vi "Run Step.vi"(8 "error in (no error)":errorcluster, 9 "result allocation":T1, 10 "parameters":T1, 11 "Step in":refnum<class "Step.lvclass">) -> (0 "error out":errorcluster, 1 "results":T1, 2 "parameter allocation":T1, 3 "Step out":refnum<class "Step.lvclass">)   [LabVIEW 2015, in "Step.lvclass"]
uses:
  Step.lvclass
  <vilib>/NI/Tag Bus/table/data table.ctl
  StepState.ctl
  Step State Enum.ctl
  Step Flow Control.ctl
  Step.lvclass/Step.ctl
  <vilib>/NI/Tag Bus/table/data table.lvlib
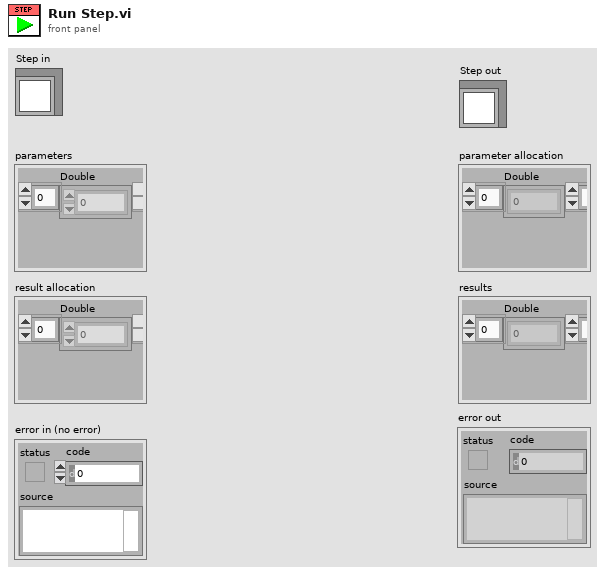
[diagram p1: front panel]
types:
  T1 = typedef "tag bus.lvlib/data table.lvlib/data table.ctl" = cluster{"Double":dbl[], "Single":sgl[], "I64":i64[], "I32":i32[], "I16":i16[], "I8":i8[], "U64":u64[], "U32":u32[], "U16":u16[], "U8":u8[], "Boolean":bool[], "String":string[], "Array of Double":cluster{"DBL Array":dbl[]}[], "Array of Single":cluster{"SGL Array":sgl[]}[], "Array of I64":cluster{"I64 Array":i64[]}[], "Array of I32":cluster{"I32 Array":i32[]}[], "Array of I16":cluster{"I16 Array":i16[]}[], "Array of I8":cluster{"I8 Array":i8[]}[], "Array of U64":cluster{"U64 Array":u64[]}[], "Array of U32":cluster{"U32 Array":u32[]}[], "Array of U16":cluster{"U16 Array":u16[]}[], "Array of U8":cluster{"U8 Array":u8[]}[], "Array of Boolean":cluster{"Boolean Array":bool[]}[], "Array of String":cluster{"String Array":string[]}[]}
  T2 = typedef "Step.lvclass/StepState.ctl" = cluster{"Step State":T3, "Flow Control":T4, "Jump Index":i32}
  T3 = typedef "Step.lvclass/Step State Enum.ctl" = enum16{"Start", "Skipped", "Timeout", "Completed", "Running", "Aborted"}
  T4 = typedef "Step.lvclass/Step Flow Control.ctl" = enum16{"Next Step", "Jump"}
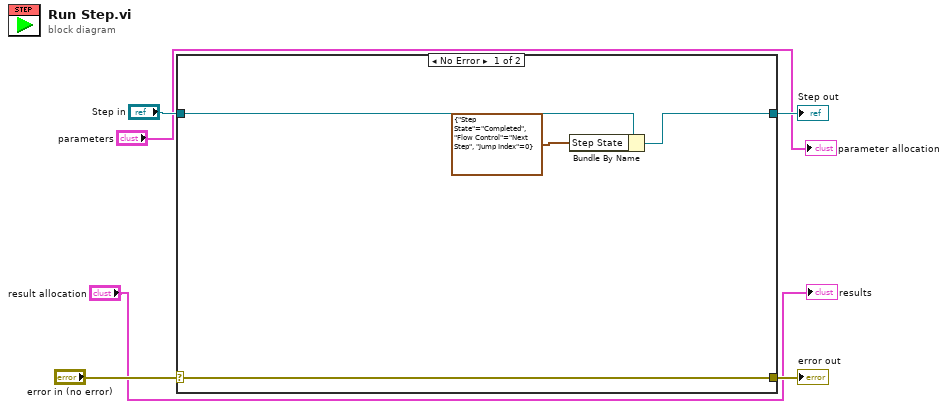
[diagram p0: block diagram]
diagram:
  n1 = case shown="No Error" "error in (no error)" {
    selector: "error in (no error)" -> [w10 w12]
    tunnel: [w10 w12] -> w5
    tunnel: [w8 w11] -> w3
    tunnel: "Step in" -> [w9 w11]
    frame No Error {
      n2 = Bundle By Name(cluster=w9, "Step State"=T2 {"Step State"=enum."Completed", "Flow Control"=enum."Next Step", "Jump Index"=0}) -> (w8:refnum<class "Step.lvclass">)
    }
    frame Error {
    }
  }
  "error out" <- w5
  "Step out" <- w3
  "parameter allocation" <- "parameters"
  "results" <- "result allocation"
